vi "cp.vi"() -> ()   [LabVIEW 2018]
uses:
  <vilib>/MediaMongrels Ltd/WebSockets/WebSockets/WebSocket Client/WebSocket Client.lvclass
  D:/software_setup/National Instruments/LabVIEW 2018/vi.lib/MediaMongrels Ltd/WebSockets/WebSockets/WebSocket/WebSocket.lvclass
panel:
  out "Data":string
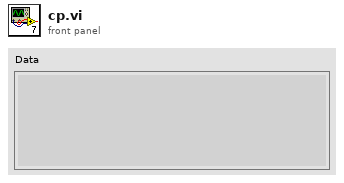
[diagram p1: front panel]
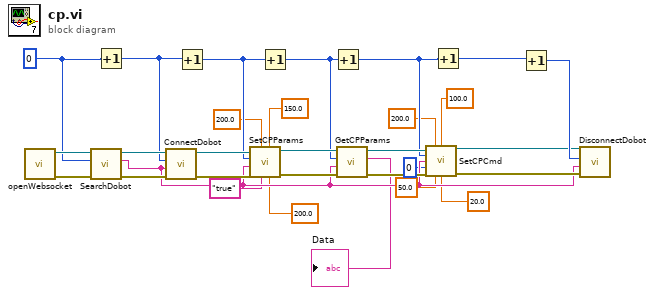
[diagram p0: block diagram]
diagram:
  w26 = 0 ("id")
  n1 = call <vilib>:"openWebsocket.vi"() -> ("error out"=w28:errorcluster, "WebSocket Client out"=w30:refnum<class "WebSocket Client.lvclass">)  [unwired: 10 in]
  n2 = call <vilib>:"SearchDobot.vi"("error in (no error)"=w28, "id"=w26, "WebSocket in"=w30) -> ("error out"=w27:errorcluster, "portName"=w11:string, "WebSocket out"=w29:refnum<class "WebSocket Client.lvclass">)  [unwired: 6 in]
  n3 = Increment(x=w26) -> (x+1=w25:i32)
  n4 = call <vilib>:"ConnectDobot.vi"("error in (no error)"=w27, "portName"=w11, "id"=w25, "WebSocket in"=w29) -> ("error out"=w18:errorcluster, "WebSocket out"=w22:refnum<class "WebSocket Client.lvclass">)  [unwired: 5 in, 1 out]
  n5 = Increment(x=w25) -> (x+1=w14:i32)
  n6 = call <vilib>:"SetCPParams.vi"("acc"=200.0, "junctionVel"=150.0, "isRealTimeTrack"="true", "targetAcc"=200.0, "error in (no error)"=w18, "portName"=w11, "id"=w14, "WebSocket in"=w22) -> ("error out"=w17:errorcluster, "WebSocket out"=w21:refnum<class "WebSocket Client.lvclass">)  [unwired: 1 in, 1 out]
  n7 = Increment(x=w14) -> (x+1=w13:i32)
  n8 = Increment(x=w13) -> (x+1=w12:i32)
  n9 = call <vilib>:"GetCPParams.vi"("error in (no error)"=w17, "portName"=w11, "id"=w13, "WebSocket in"=w21) -> ("error out"=w16:errorcluster, "Data"=→"Data":string, "WebSocket out"=w20:refnum<class "WebSocket Client.lvclass">)  [unwired: 5 in]
  n10 = call <vilib>:"SetCPCmd.vi"("WebSocket in"=w20, "x"=200.0, "y"=100.0, "id"=w12, "portName"=w11, "cpMode"=0, "error in (no error)"=w16, "z"=50.0, "power"=20.0) -> ("WebSocket out"=w19:refnum<class "WebSocket Client.lvclass">, "error out"=w15:errorcluster)  [unwired: 4 in, 1 out]
  n11 = Increment(x=w12) -> (x+1=w23:i32)
  n12 = Increment(x=w23) -> (x+1=w24:i32)
  n13 = call <vilib>:"DisconnectDobot.vi"("error in (no error)"=w15, "portName"=w11, "id"=w24, "WebSocket in"=w19) -> ()  [unwired: 5 in, 3 out]
